vi "Sort ID table.vi"(9 "ID":u32[](array[numeric]), 10 "Family":u32[](array[numeric]), 11 "Name":string[](array[string])) -> (1 "Sorted ID":u32[](array[numeric]), 2 "Sorted Fam":u32[](array[numeric]), 3 "Sorted name":string[](array[string]))   [LabVIEW 2019, in "LINXx.lvlib"]
uses:
  38b152e7-4196-4758-a2f3-022f4908c20a.vi
  bcb42c65-d14c-4812-aee0-e974f35f8927.vi
  LINXx.lvlib
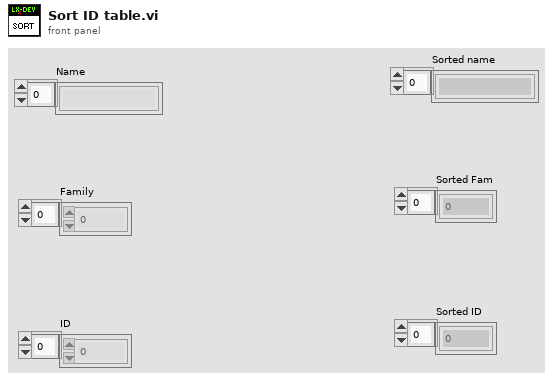
[diagram p1: front panel]
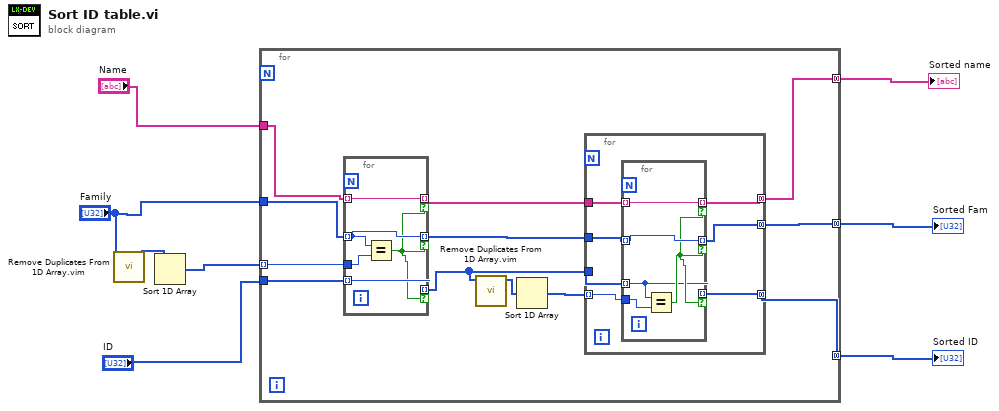
[diagram p0: block diagram]
diagram:
  n1 = call "Remove Duplicates From 1D Array.vim"("array"="Family") -> ("array with duplicates removed"=w5:u32[])  [unwired: 10 in]
  n2 = Sort 1D Array(array=w5) -> (sorted array=w4:u32[])
  n3 = for {
    tunnel: "Family" -> [w20]
    tunnel: "Name" -> [w19]
    tunnel: "ID" -> [w18]
    tunnel: w4 -> [w17] mode=indexing
    tunnel: [w12] -> w3 mode=concatenating
    tunnel: [w11] -> w2 mode=concatenating
    tunnel: [w10] -> w1 mode=concatenating
    n4 = for {
      tunnel: w20 -> [w34] mode=indexing
      tunnel: w19 -> [w36] mode=indexing
      tunnel: w18 -> [w35] mode=indexing
      tunnel: w17 -> [w37]
      tunnel: [w36] -> w15 mode=indexing if=w33
      tunnel: [w35] -> w9 mode=indexing if=w33
      tunnel: [w34] -> w14 mode=indexing if=w33
      n5 = Equal?(x=w34, y=w37) -> (x = y?=w33:bool)
    }
    n6 = call "Remove Duplicates From 1D Array.vim"("array"=w9) -> ("array with duplicates removed"=w16:u32[])  [unwired: 10 in]
    n7 = Sort 1D Array(array=w16) -> (sorted array=w13:u32[])
    n8 = for {
      tunnel: w15 -> [w27]
      tunnel: w14 -> [w26]
      tunnel: w13 -> [w25] mode=indexing
      tunnel: [w24] -> w12 mode=concatenating
      tunnel: [w23] -> w11 mode=concatenating
      tunnel: [w22] -> w10 mode=concatenating
      tunnel: w9 -> [w21]
      n9 = for {
        tunnel: w26 -> [w31] mode=indexing
        tunnel: w27 -> [w32] mode=indexing
        tunnel: w21 -> [w28] mode=indexing
        tunnel: w25 -> [w29]
        tunnel: [w32] -> w24 mode=indexing if=w30
        tunnel: [w28] -> w22 mode=indexing if=w30
        tunnel: [w31] -> w23 mode=indexing if=w30
        n10 = Equal?(x=w28, y=w29) -> (x = y?=w30:bool)
      }
    }
  }
  "Sorted name" <- w3
  "Sorted Fam" <- w2
  "Sorted ID" <- w1
